vi "Write_Data.vi"(8 "error in (no error)":errorcluster caption="entrée d'erreur (pas d'erreur)", 10 "Data_To_Write":string, 11 "Class Instrument Firebase Altyor en entrée":refnum<class "Class Instrument Firebase Altyor.lvclass">) -> (0 "error out":errorcluster caption="sortie d'erreur", 3 "Class Instrument Firebase Altyor en sortie":refnum<class "Class Instrument Firebase Altyor.lvclass">)   [LabVIEW 2020, in "Library Instrument & Equipement.lvlib" / "Library Instruments.lvlib" / "Class Instrument Firebase Altyor.lvclass"]
uses:
  Class Instrument Firebase Altyor.lvclass
  Class Instrument Firebase Altyor.lvclass/Class Instrument Firebase Altyor.ctl
  Firebase/Source/Firebase Altyor/Firebase Altyor.lvclass
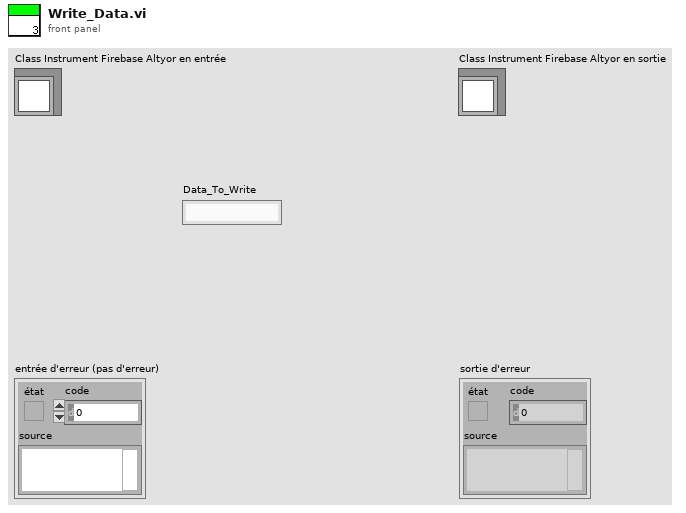
[diagram p1: front panel]
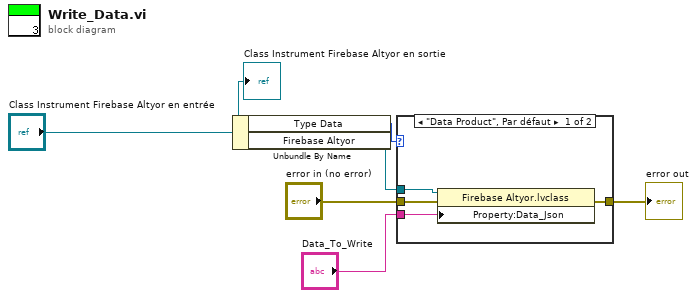
[diagram p0: block diagram]
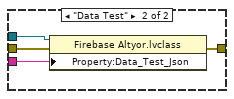
[diagram p2: hidden frame]
diagram:
  n1 = Unbundle By Name("Class Instrument Firebase Altyor en entrée") -> ("Type Data"=w6:enum16{"Data Product", "Data Test"}, "Firebase Altyor"=w5:refnum<class "Firebase Altyor.lvclass">)
  n2 = case shown="\"Data Product\", Par défaut" w6 {
    tunnel: "error in (no error)" -> [w9 w13]
    tunnel: w5 -> [w10 w14]
    tunnel: "Data_To_Write" -> [w7 w12]
    tunnel: [w8 w11] -> w1
    frame "Data Product", Default {
      n3 = property class="Firebase Altyor.lvclass"(reference=w10, error in=w9, "Property:Data_Json"=w7) -> (error out=w8:errorcluster)  [unwired: 1 out]
    }
    frame "Data Test" {
      n4 = property class="Firebase Altyor.lvclass"(reference=w14, error in=w13, "Property:Data_Test_Json"=w12) -> (error out=w11:errorcluster)  [unwired: 1 out]
    }
  }
  "error out" <- w1
  "Class Instrument Firebase Altyor en sortie" <- "Class Instrument Firebase Altyor en entrée"
